vi "DrawCrossHair.vi"(8 "error in (no error)":errorcluster, 10 "Point":cluster{"X":i32, "Y":i32}, 11 "Image In":T1) -> (0 "error out":errorcluster, 3 "Image Out":T1)   [LabVIEW 2017]
doc: "Use this template to build a VI to use as a subVI."
uses:
  <vilib>/vision/Image Controls.llb/IMAQ Image.ctl
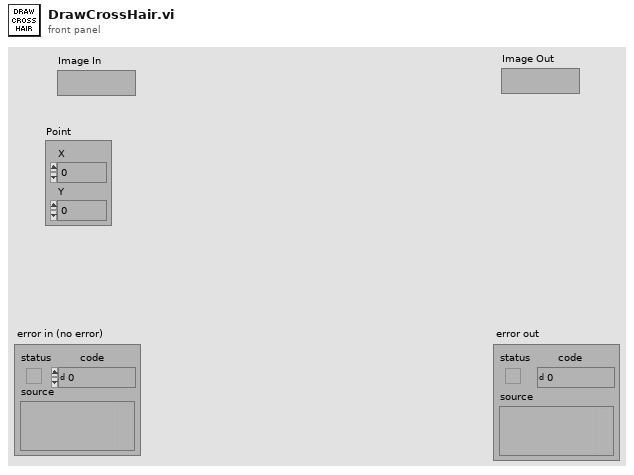
[diagram p1: front panel]
types:
  T1 = typedef "IMAQ Image.ctl" = refnum<image>
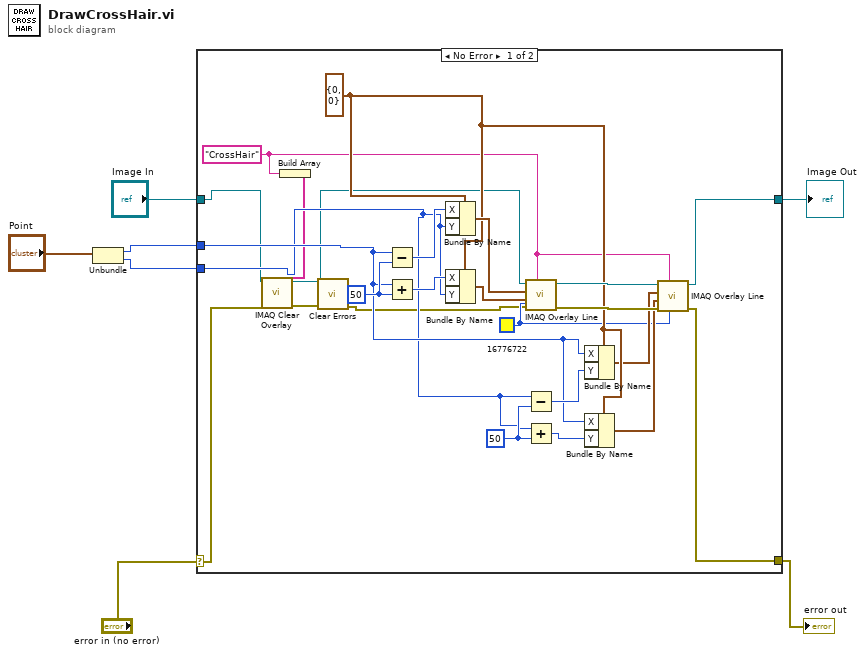
[diagram p0: block diagram]
diagram:
  n1 = Unbundle("Point") -> ("X"=w2:i32, "Y"=w1:i32)
  n2 = case shown="No Error" "error in (no error)" {
    selector: "error in (no error)" -> [w14 w34]
    tunnel: [w19 w34] -> w6
    tunnel: [w18 w33] -> w5
    tunnel: "Image In" -> [w13 w33]
    tunnel: w2 -> [w16 _]
    tunnel: w1 -> [w15 _]
    frame No Error {
      w25 = 50
      w30 = 50
      w24 = cluster{"X":i32, "Y":i32} {"X"=0, "Y"=0} ("Start Point")
      w11 = "CrossHair" ("Group")
      w17 = u32 16776722 ("Color")
      n3 = Build Array(w11) -> (w10:string[])
      n4 = call "IMAQ Clear Overlay"("Groups"=w10, "error in (no error)"=w14, "Image"=w13) -> ("error out"=w9:errorcluster, "Image Out"=w12:T1)  [unwired: 7 in]
      n5 = call <vilib>:"Clear Errors.vi"("error in (no error)"=w9) -> ("error out"=w8:errorcluster)  [unwired: 5 in, 1 out]
      n6 = Subtract(x=w16, y=w30) -> (x-y=w32:i32)
      n7 = Add(x=w16, y=w30) -> (x+y=w29:i32)
      n8 = Bundle By Name(cluster=w24, "X"=w32, "Y"=w15) -> (w31:cluster{"X":i32, "Y":i32})
      n9 = Bundle By Name(cluster=w24, "X"=w29, "Y"=w15) -> (w28:cluster{"X":i32, "Y":i32})
      n10 = call "IMAQ Overlay Line"("Color"=w17, "Group"=w11, "error in (no error)"=w8, "End Point"=w28, "Start Point"=w31, "Image"=w12) -> ("error out"=w27:errorcluster, "Image Out"=w26:T1)  [unwired: 4 in]
      n11 = Subtract(x=w15, y=w25) -> (x-y=w22:i32)
      n12 = Add(x=w15, y=w25) -> (x+y=w23:i32)
      n13 = Bundle By Name(cluster=w24, "X"=w16, "Y"=w22) -> (w20:cluster{"X":i32, "Y":i32})
      n14 = Bundle By Name(cluster=w24, "X"=w16, "Y"=w23) -> (w21:cluster{"X":i32, "Y":i32})
      n15 = call "IMAQ Overlay Line"("Color"=w17, "Group"=w11, "error in (no error)"=w27, "End Point"=w21, "Start Point"=w20, "Image"=w26) -> ("error out"=w19:errorcluster, "Image Out"=w18:T1)  [unwired: 4 in]
    }
    frame Error {
    }
  }
  "error out" <- w6
  "Image Out" <- w5
